vi "getU8.vi"(7 "offset":i32, 8 "String":string) -> (3 "value":i32)   [LabVIEW 2013]
doc: "Get an U8 from string at offset"
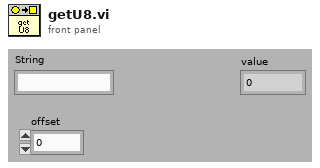
[diagram p1: front panel]
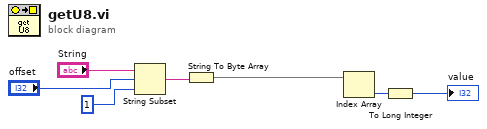
[diagram p0: block diagram]
diagram:
  n1 = String Subset(string="String", offset (0)="offset", length (rest)=1 ("length (rest)")) -> (substring=w4:string)
  n2 = String To Byte Array(string=w4) -> (unsigned byte array=w1:u8[])
  n3 = Index Array(array=w1) -> (element=w3:u8)  [unwired: 1 in]
  n4 = To Long Integer(number=w3) -> (32bit integer=→"value":i32)
